vi "prepDO_res.vi"() -> ()   [LabVIEW 2015]
uses:
  <vilib>/DAQmx/write.llb/DAQmx Write (Digital 1D Wfm NChan NSamp).vi
  waveforms/usedDOindepofwf.vi
  Objects/waveformsDObuffer.vi
  <vilib>/DAQmx/create/channels.llb/DAQmx Create Channel (DO-Digital Output).vi
  <vilib>/DAQmx/configure/timing.llb/DAQmx Timing (Sample Clock).vi
  <vilib>/Waveform/DWDTOps.llb/DWDT Uncompress Digital.vi
  <vilib>/DAQmx/miscellaneous.llb/DAQmx Fill In Error Info.vi
panel:
  in  "error in":errorcluster
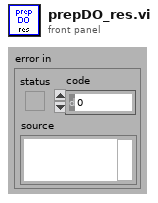
[diagram p1: front panel]
types:
  T1 = cluster{"StageS":i32, "StageL":i32, "currmeas data dir":path, "image OD":u16, "contour OD":u16, "point OD":u16, "AOlines":tag[], "AIlines":tag[], "CI lines":tag[], "DO lines":tag[], "AO names":string[], "CI names":string[], "AI names":string[], "DO names":string[], "CIextensions":string[], "AIextensions":string[], "Voltage to Ygalvo":i32, "Voltage to Xgalvo":i32, "Voltage to patch":i32, "640 shutter":i32, "2P shutter":i32, "LT timestamp":u32, "Vp":i32, "Ip":i32, "camera trigger":i32, "master data dir":path, "voltage to Zpos":i32, "Vto2P":i32, "640 AO":i32, "488 AO":i32, "532 AO":i32, "640TTL":u32, "488TTL":u32, "532TTL":u32}
  T2 = typedef "LVRectTypeDef.ctl" = cluster{"Left":i16, "Top":i16, "Right":i16, "Bottom":i16}
  T3 = cluster{"Xpixels":i32, "Vxminref":dbl, "Vxmaxref":dbl, "P":dbl, "Ypixels":i32, "Vyminref":dbl, "Vymaxref":dbl, "srate":sgl, "sAOxy":i32, "timeout":dbl, "type":string, "date":string, "time":string, "Colormap":u16, "Drawing Mode":u16, "Scanning Mode":u16, "square pixels":bool, "square matrix":bool, "Xpixels Img":i32, "Vx-min Img":dbl, "VX-max Img":dbl, "Ypixels Img":i32, "Vy-min Img":dbl, "Vy-max Img ":dbl, "Angle Img":dbl, "autoshutter":bool, "finite":bool, "cont":bool, "wavdet":bool, "measpoints":i32, "avpp":i32, "bufferAO":i32, "bufferAI":i32, "starttick":u32, "waveform":path, "Vx-ref":dbl, "Vy-ref":dbl, "refreshrate":dbl, "refreshbuffer":i32, "tt_cycles":i32, "motorref":refnum<k7>, "mirrorswitch":refnum<k7>, "sample mode":i32, "maxbufferAI":i32, "srateAODO":sgl, "bin":sgl, "Pel":sgl, "Angle draw":dbl, "srate Img":sgl, "ROIimg_plotbounds":T2, "auto OD":bool, "ODfilt":u16, "aAI":i32[], "aCI":i32[], "aAO":u32[], "aDO":u32[], "refwfsize":dbl, "Lifetime":bool, "Vz-Img":dbl, "Vz-ref":dbl, "Vz-reset":dbl, "AIoverride":bool}
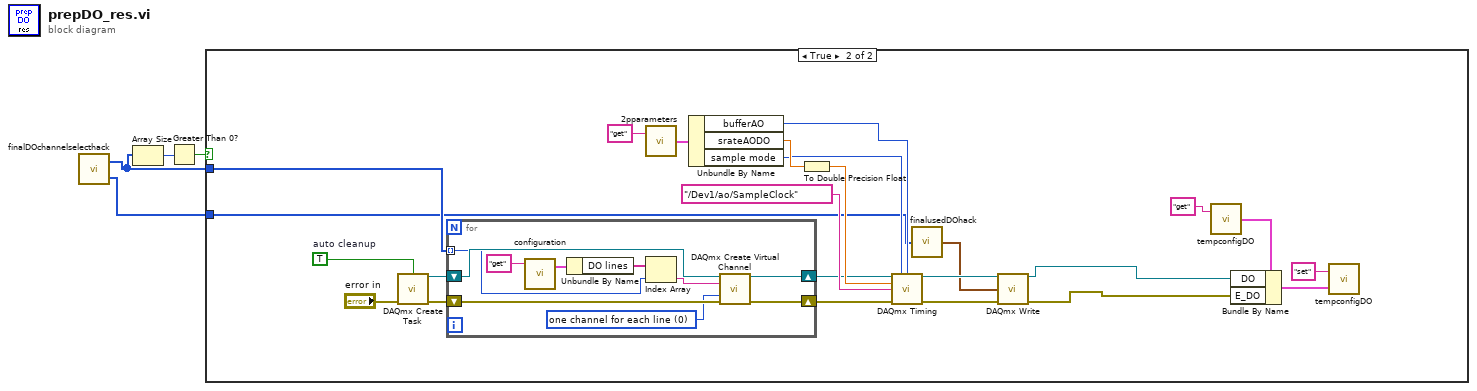
[diagram p0: block diagram]
diagram:
  n1 = call "finalDOchannelselecthack.vi"() -> ("usedDO"=w2:u32[], "presorted indices"=w1:u32[])  [unwired: 1 in]
  n2 = Array Size(array=w2) -> (size(s)=w3:i32)
  n3 = Greater Than 0?(x=w3) -> (x > 0?=w4:bool)
  n4 = case shown="True" w4 {
    tunnel: w2 -> [_ w15]
    tunnel: w1 -> [_ w5]
    frame False {
    }
    frame True {
      w27 = TRUE  # auto cleanup
      n5 = call <vilib>:"DAQmx Create Task.vi"("auto cleanup"=w27, "error in"="error in") -> ("task out"=w28:refnum<k21>, "error out"=w26:errorcluster)  [unwired: 12 in]
      n6 = for {
        shift-right: [w30] -> w18
        shift-left: w26 -> [w37]
        tunnel: w15 -> [w34] mode=indexing
        shift-right: [w31] -> w19
        shift-left: w28 -> [w38]
        w29 = 0 items=["one channel for each line", "one channel for all lines"] ("line grouping")
        n7 = call "configuration.vi"("command"="get") -> ("config out"=w36:T1)  [unwired: 2 in, 1 out]
        n8 = Unbundle By Name(w36) -> ("DO lines"=w33:tag[])
        n9 = Index Array(array=w33, index=w34) -> (element=w32:tag)
        n10 = call-poly <vilib>:"DAQmx Create Virtual Channel.vi"("task in"=w38, "lines"=w32, "line grouping"=w29, "error in"=w37) -> ("task out"=w31:refnum<k21>, "error out"=w30:errorcluster)  [unwired: 10 in]
      }
      n11 = call "2pparameters.vi"("command"="get") -> ("params out"=w24:T3)  [unwired: 1 in]
      n12 = Unbundle By Name(w24) -> ("bufferAO"=w17:i32, "srateAODO"=w20:sgl, "sample mode"=w16:i32)
      n13 = To Double Precision Float(number=w20) -> (double precision float=w22:dbl)
      n14 = call-poly <vilib>:"DAQmx Timing.vi"("task/channels in"=w19, "sample mode"=w16, "samples per channel"=w17, "rate"=w22, "source"=tag "/Dev1/ao/SampleClock", "error in"=w18) -> ("task out"=w14:refnum<k21>, "error out"=w13:errorcluster)  [unwired: 1 in, 7 out]
      n15 = call "finalusedDOhack.vi"("presorted indices"=w5) -> ("DO"=w8:digitalwaveform[])
      n16 = call-poly <vilib>:"DAQmx Write.vi"("task/channels in"=w14, "data"=w8, "error in"=w13) -> ("task out"=w7:refnum<k21>, "error out"=w6:errorcluster)  [unwired: 10 in, 1 out]
      n17 = call "tempconfigDO.vi"("command"="get") -> ("Temp Config out"=w11:cluster{"DO":refnum<k21>, "E_DO":errorcluster})  [unwired: 1 in]
      n18 = Bundle By Name(cluster=w11, "DO"=w7, "E_DO"=w6) -> (w9:cluster{"DO":refnum<k21>, "E_DO":errorcluster})
      n19 = call "tempconfigDO.vi"("Temp Config in"=w9, "command"="set") -> ()  [unwired: 1 out]
    }
  }
